vi "Plot_Individual_folder.vi"() -> ()   [LabVIEW 2019]
uses:
  <vilib>/Utility/file.llb/Read Delimited Spreadsheet (DBL).vi
panel:
  in  "stop":bool
  out "Spectrum Data":cluster{"all rows":dbl[], "all rows":dbl[]}(graph) caption="XY Graph - Dark"
  in  "Files":i32(listbox)
  in  "Folder Path":path
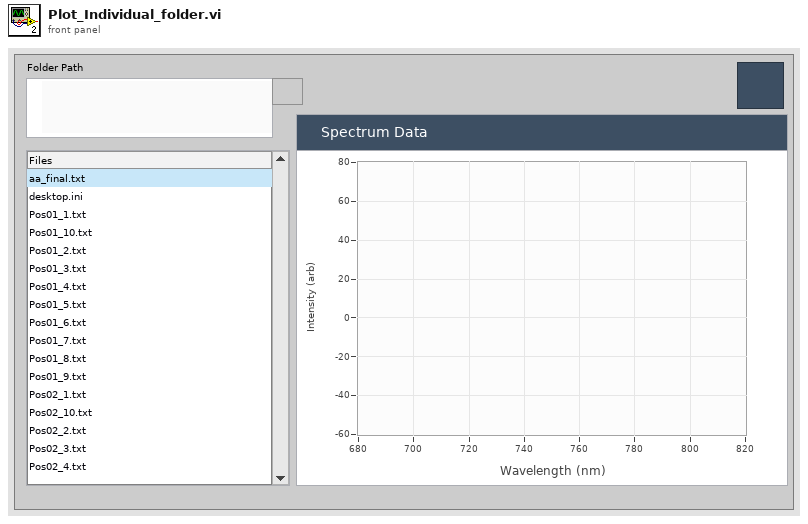
[diagram p1: front panel]
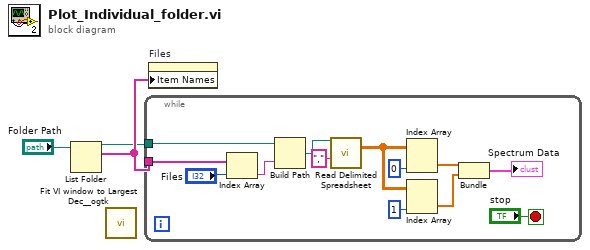
[diagram p0: block diagram]
diagram:
  n1 = List Folder(path="Folder Path") -> (path out=w1:path, filenames=w2:string[])  [unwired: 3 in, 2 out]
  n2 = call <userlib>:"Fit VI window to Largest Dec__ogtk.vi"() -> ()  [unwired: 6 in, 2 out]
  n3 = while {
    tunnel: w2 -> [w16]
    tunnel: w1 -> [w14]
    stop <- "stop" stop-if-true
    n4 = Index Array(array=w16, index="Files") -> (element=w13:string)
    n5 = Build Path(base path=w14, name or relative path=w13) -> (appended path=w12:path)
    n6 = call-poly <vilib>:"Read Delimited Spreadsheet.vi"("file path (dialog if empty)"=w12, "delimiter (\\t)"="," ("delimiter (\\t)")) -> ("all rows"=w10:dbl[][])  [unwired: 8 in, 5 out]
    n7 = Index Array(array=w10, index (col)=0 ("disabled index (col)")) -> (element=w7:dbl[])  [unwired: 1 in]
    n8 = Index Array(array=w10, index (col)=1 ("disabled index (col)")) -> (element=w6:dbl[])  [unwired: 1 in]
    n9 = Bundle("all rows"=w7, "all rows"=w6) -> (→"Spectrum Data":cluster{"all rows":dbl[], "all rows":dbl[]})  [unwired: 1 in]
  }
  n10 = property on="Files" class="LstBox (strict)"("Item Names"=w2) -> ()  [unwired: 2 in, 2 out]
